vi "Main.vi"() -> ()   [LabVIEW 2022 SP3]
uses:
  <vilib>/Analysis/baseanly.llb/Mean (DBL).vi
  <vilib>/Analysis/NI_AALBase.lvlib
panel:
  in  "Calibration points":T1(array[ring])
  out "Results:":string[][](table)
  in  "Voltage [V] (max. 3.5V)":string
  in  "Confirm initialization":bool
  in  "100K FILTER":u16(ring) items=["FILTER ON", "FILTER OFF"]
  in  "IMPEDANCE [Ohm]":u16(ring) items=["50", "1M"]
  in  "COUPLING":u16(ring) items=["AC", "DC"]
  in  "counter Agilent 53131A - GPIB  [10]":string="1"
  in  "Number of measurements for each calibration point:[max 20]":i32=5
  in  "oscilloscope  Siglent SDS1102X+":refnum<visa-resource-name>="COM1"
  out "Current state:":enum16{"Init", "Measure", "Wait", "End"}(ring)
  in  "Start measuring":bool
  in  "STOP button":bool
  in  "generator Agilent 33220A":refnum<visa-resource-name>="COM1"
  # "Input settings:"
  # "Measuring:"
  # "Measurement settings:"
  # "Generator settings:"
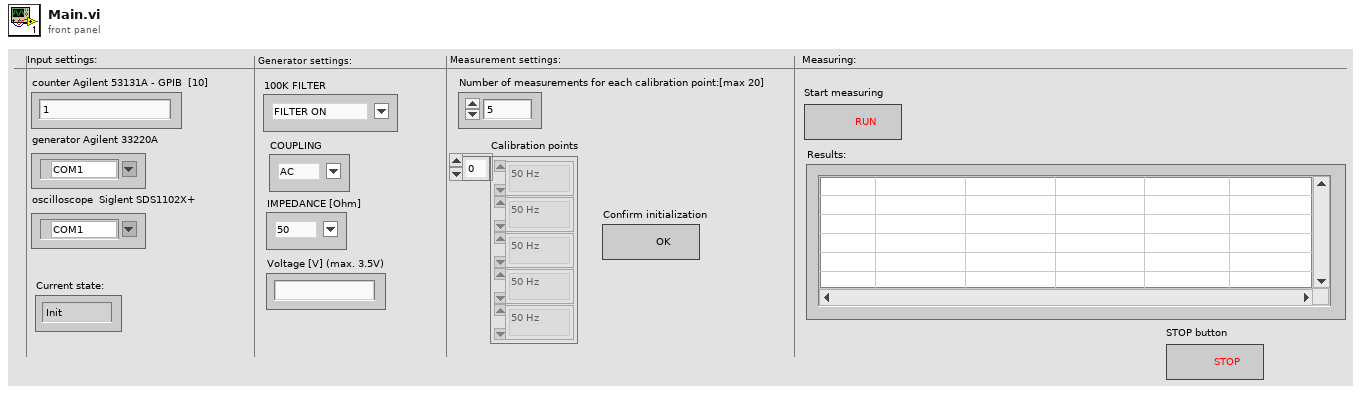
[diagram p1: front panel]
types:
  T1 = enum16{"50 Hz", "1 kHz", "5 kHz", "20 kHz", "50 kHz", "100 kHz"}[]
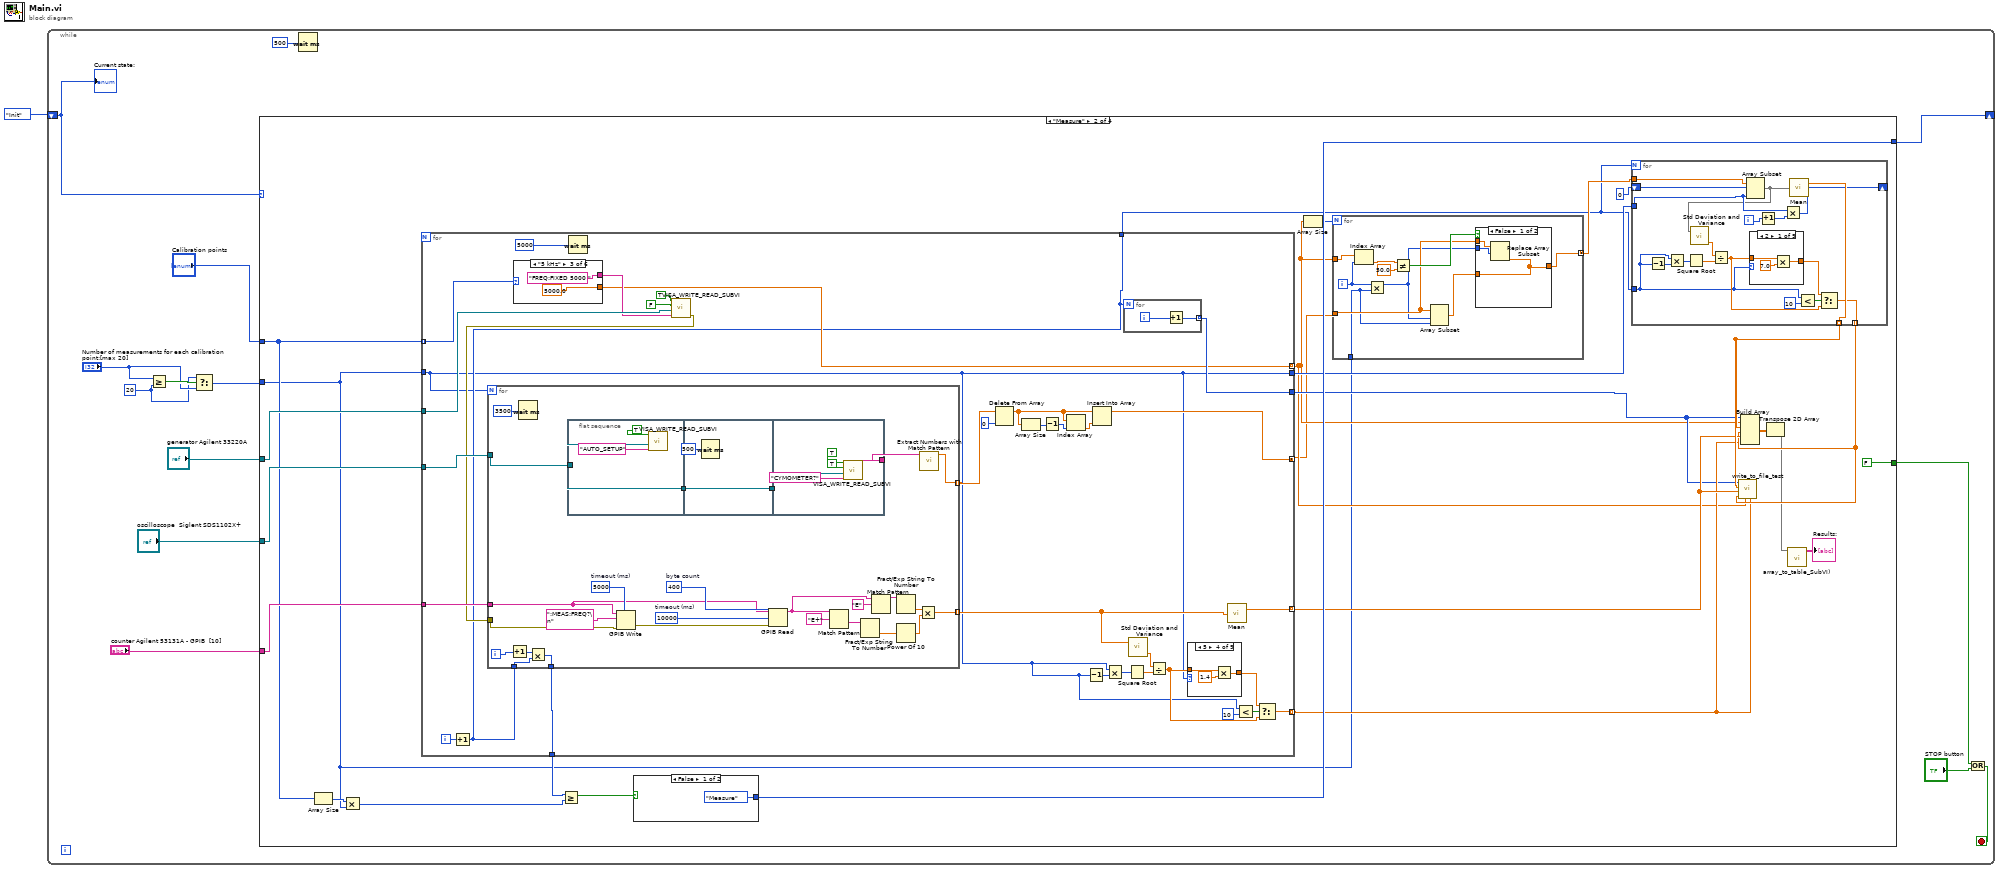
[diagram p0: block diagram]
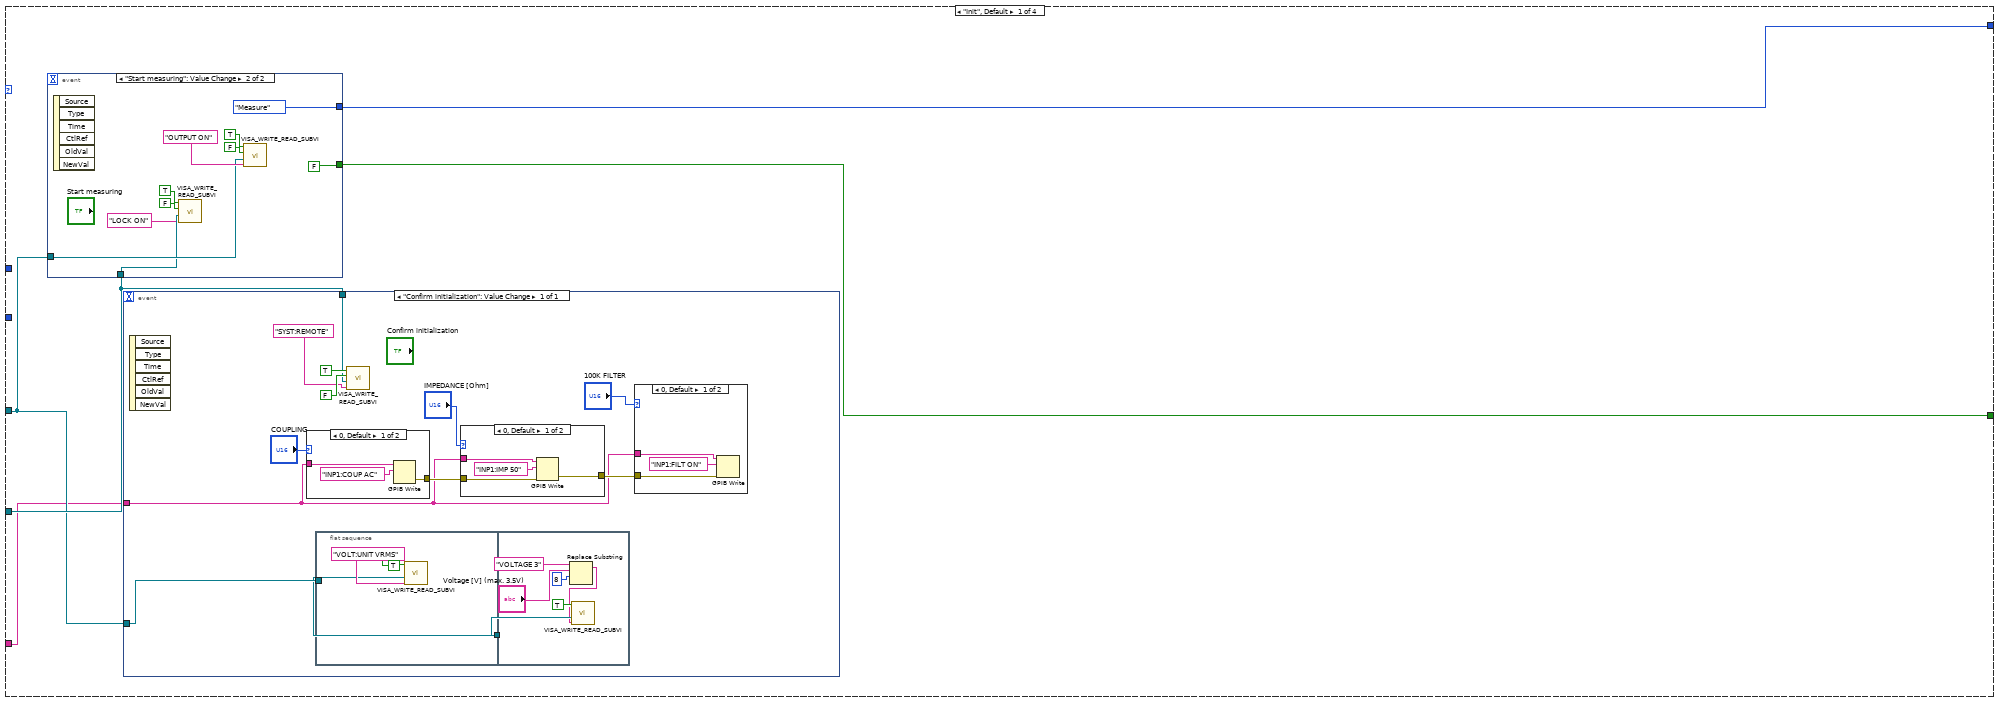
[diagram p2: hidden frame]
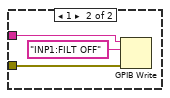
[diagram p3: hidden frame]
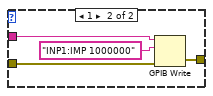
[diagram p4: hidden frame]
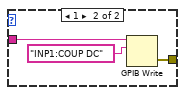
[diagram p5: hidden frame]
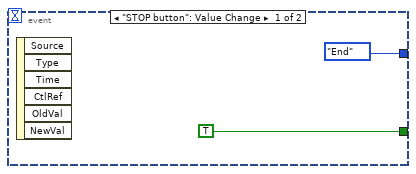
[diagram p6: hidden frame]
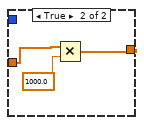
[diagram p7: hidden frame]
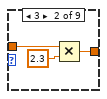
[diagram p8: hidden frame]
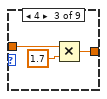
[diagram p9: hidden frame]
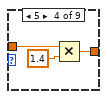
[diagram p10: hidden frame]
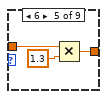
[diagram p11: hidden frame]
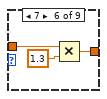
[diagram p12: hidden frame]
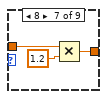
[diagram p13: hidden frame]
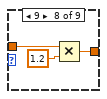
[diagram p14: hidden frame]
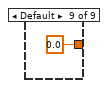
[diagram p15: hidden frame]
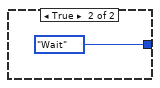
[diagram p16: hidden frame]
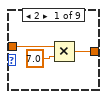
[diagram p17: hidden frame]
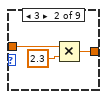
[diagram p18: hidden frame]
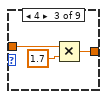
[diagram p19: hidden frame]
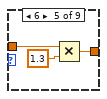
[diagram p20: hidden frame]
diagram:
  n1 = while {
    shift-right: [w4] -> _
    shift-left: enum16{"Init", "Measure", "Wait", "End"}."Init" -> [w14]
    stop <- w5 stop-if-true
    w9 = 20 ("y")
    n2 = Greater Or Equal?(x="Number of measurements for each calibration point:[max 20]", y=w9) -> (x >= y?=w11:bool)
    n3 = Select(t=w9, s=w11, f="Number of measurements for each calibration point:[max 20]") -> (s? t:f=w8:i32)
    n4 = case shown="\"Measure\"" w14 {
      tunnel: [w20 w93 enum16{"Init", "Measure", "Wait", "End"}."Init" enum16{"Init", "Measure", "Wait", "End"}."Init"] -> w4
      tunnel: [w16 FALSE ("stop") FALSE ("stop") TRUE ("stop")] -> w6
      tunnel: "generator Agilent 33220A" -> [w18 w98 _ _]
      tunnel: "Calibration points" -> [_ w95 _ _]
      tunnel: "oscilloscope  Siglent SDS1102X+" -> [w19 w97 _ _]
      tunnel: w8 -> [_ w77 _ _]
      tunnel: "counter Agilent 53131A - GPIB  [10]" -> [w17 w96 _ _]
      frame "Init", Default {
        n5 = event shown="[1] \"Start measuring\": Value Change" {
          selector: _ -> [_ _]
          dyn-events: _ -> [_ _]
          timeout: _ -> [_ _]
          tunnel: [enum16{"Init", "Measure", "Wait", "End"}."End" enum16{"Init", "Measure", "Wait", "End"}."Measure"] -> w20
          tunnel: [TRUE ("stop") FALSE ("Boolean")] -> w16
          tunnel: w18 -> [_ w71]
          tunnel: w19 -> [_ w68]
          event "STOP button": Value Change {
            n6 = event-data() -> ()  [unwired: 1 in, 6 out]
          }
          event "Start measuring": Value Change {
            n7 = event-data() -> ()  [unwired: 1 in, 6 out]
            n8 = call "VISA_WRITE_READ_SUBVI.vi"("Command"="LOCK ON", "VISA resource name"=w68, "Read 2"=FALSE ("Read"), "Write 2"=TRUE ("Write")) -> ()  [unwired: 3 in, 2 out]
            n9 = call "VISA_WRITE_READ_SUBVI.vi"("Command"="OUTPUT ON", "VISA resource name"=w71, "Read 2"=FALSE ("Read"), "Write 2"=TRUE ("Write")) -> ()  [unwired: 3 in, 2 out]
          }
        }
        n10 = event shown="[0] \"Confirm initialization\": Value Change" {
          selector: _ -> [_]
          dyn-events: _ -> [_]
          timeout: _ -> [_]
          tunnel: w19 -> [w30]
          tunnel: w18 -> [w22]
          tunnel: w17 -> [w23]
          event "Confirm initialization": Value Change {
            n11 = event-data() -> ()  [unwired: 1 in, 6 out]
            n12 = case shown="0, Default" "COUPLING" {
              tunnel: w23 -> [w58 w61]
              tunnel: [w56 w59] -> w28
              frame 0, Default {
                n13 = GPIB Write(0:w58, 1:"INP1:COUP AC" ("Command")) -> (6:w56:errorcluster)  [unwired: 3 in, 1 out]
              }
              frame 1 {
                n14 = GPIB Write(0:w61, 1:"INP1:COUP DC" ("Command")) -> (6:w59:errorcluster)  [unwired: 3 in, 1 out]
              }
            }
            n15 = flat-sequence {
              tunnel: w22 -> [w33]
              tunnel: [w33] -> w21
              tunnel: w21 -> [w40]
              frame #0 {
                n16 = call "VISA_WRITE_READ_SUBVI.vi"("Command"="VOLT:UNIT VRMS", "VISA resource name"=w33, "Write 2"=TRUE) -> ()  [unwired: 4 in, 2 out]
              }
              frame #1 {
                n17 = Replace Substring(3:8 ("offset (0)"), 4:"Voltage [V] (max. 3.5V)", 5:"VOLTAGE 3" ("Command")) -> (1:w36:string)  [unwired: 1 in, 1 out]
                n18 = call "VISA_WRITE_READ_SUBVI.vi"("Command"=w36, "VISA resource name"=w40, "Write 2"=TRUE) -> ()  [unwired: 4 in, 2 out]
              }
            }
            n19 = call "VISA_WRITE_READ_SUBVI.vi"("Command"="SYST:REMOTE", "VISA resource name"=w30, "Read 2"=FALSE ("Read"), "Write 2"=TRUE ("Write")) -> ()  [unwired: 3 in, 2 out]
            n20 = case shown="0, Default" "IMPEDANCE [Ohm]" {
              tunnel: w23 -> [w51 w53]
              tunnel: w28 -> [w49 w54]
              tunnel: [w48 w55] -> w27
              frame 0, Default {
                n21 = GPIB Write(0:w51, 1:"INP1:IMP 50" ("Command"), 3:w49) -> (6:w48:errorcluster)  [unwired: 2 in, 1 out]
              }
              frame 1 {
                n22 = GPIB Write(0:w53, 1:"INP1:IMP 1000000" ("Command"), 3:w54) -> (6:w55:errorcluster)  [unwired: 2 in, 1 out]
              }
            }
            n23 = case shown="0, Default" "100K FILTER" {
              tunnel: w23 -> [w43 w46]
              tunnel: w27 -> [w42 w45]
              frame 0, Default {
                n24 = GPIB Write(0:w43, 1:"INP1:FILT ON" ("data"), 3:w42) -> ()  [unwired: 2 in, 2 out]
              }
              frame 1 {
                n25 = GPIB Write(0:w46, 1:"INP1:FILT OFF" ("data"), 3:w45) -> ()  [unwired: 2 in, 2 out]
              }
            }
          }
        }
      }
      frame "Measure" {
        n26 = Array Size(array=w95) -> (size(s)=w94:i32)
        n27 = Multiply(x=w94, y=w77) -> (x*y=w90:i32)
        n28 = for {
          tunnel: w98 -> [w183]
          tunnel: w95 -> [w178] mode=indexing
          tunnel: w77 -> [w161]
          tunnel: w97 -> [w181]
          tunnel: w96 -> [w180]
          tunnel: [w177] -> w85 mode=indexing
          tunnel: [w175] -> w91
          tunnel: [w164] -> w79 mode=concatenating
          tunnel: [w161] -> w89
          tunnel: [w174] -> w83 mode=indexing
          tunnel: [w172] -> w80 mode=indexing
          tunnel: [w173] -> w82
          tunnel: [w163] -> w76
          i -> [w162]
          n29 = Increment(x=w162) -> (x+1=w163:i32)
          n30 = case shown="\"5 kHz\"" w178 {
            tunnel: ["FREQ:FIXED 50 " ("Command") "FREQ:FIXED 1000 " ("Command") "FREQ:FIXED 5000 " ("Command") "FREQ:FIXED 20000 " ("Command") "FREQ:FIXED 50000 " ("Command") "FREQ:FIXED 100000" ("Command")] -> w182
            tunnel: [50.0 1000.0 5000.0 20000.0 50000.0 100000.0] -> w172
            frame "50 Hz", Default {
            }
            frame "1 kHz" {
            }
            frame "5 kHz" {
            }
            frame "20 kHz" {
            }
            frame "50 kHz" {
            }
            frame "100 kHz" {
            }
          }
          n31 = Wait (ms)(milliseconds to wait=u32 5000) -> ()  [unwired: 1 out]
          n32 = call "VISA_WRITE_READ_SUBVI.vi"("Command"=w182, "VISA resource name"=w183, "Read 2"=FALSE ("Read"), "Write 2"=TRUE ("Write")) -> ("error out"=w179:errorcluster)  [unwired: 3 in, 1 out]
          n33 = for {
            N: w161 -> [_]
            tunnel: w181 -> [w196]
            tunnel: w180 -> [w216]
            tunnel: [w200] -> w171 mode=indexing
            tunnel: [w212] -> w176 mode=indexing
            tunnel: w179 -> [w215]
            tunnel: w163 -> [w207]
            tunnel: [w201] -> w175
            i -> [w206]
            w217 = 10000  # timeout (ms)
            w219 = 400  # byte count
            w218 = 5000  # timeout (ms)
            n34 = Increment(x=w206) -> (x+1=w205:i32)
            n35 = Wait (ms)(milliseconds to wait=u32 3500) -> ()  [unwired: 1 out]
            n36 = Multiply(x=w205, y=w207) -> (x*y=w201:i32)
            n37 = flat-sequence {
              tunnel: w196 -> [w222]
              tunnel: [w222] -> w198
              tunnel: w198 -> [w225]
              tunnel: [w225] -> w197
              tunnel: [w228] -> w199
              tunnel: w197 -> [w227]
              frame #0 {
                n38 = call "VISA_WRITE_READ_SUBVI.vi"("Command"="AUTO_SETUP", "VISA resource name"=w222, "Write 2"=TRUE) -> ()  [unwired: 4 in, 2 out]
              }
              frame #1 {
                n39 = Wait (ms)(milliseconds to wait=u32 500) -> ()  [unwired: 1 out]
              }
              frame #2 {
                n40 = call "VISA_WRITE_READ_SUBVI.vi"("Command"="CYMOMETER?", "VISA resource name"=w227, "Read 2"=TRUE, "Write 2"=TRUE) -> ("Response"=w228:string)  [unwired: 3 in, 1 out]
              }
            }
            n41 = GPIB Write(0:w216, 1:":MEAS:FREQ?\n" ("Characters to Write"), 3:w215, 4:w218) -> (6:w221:errorcluster)  [unwired: 1 in, 1 out]
            n42 = GPIB Read(0:w216, 1:w219, 3:w221, 4:w217) -> (5:w204:string)  [unwired: 1 in, 2 out]
            n43 = Match Pattern(string=w204, regular expression="E+") -> (after substring=w213:string)  [unwired: 1 in, 3 out]
            n44 = Fract/Exp String To Number(string=w213) -> (number=w210:dbl)  [unwired: 3 in, 1 out]
            n45 = Match Pattern(string=w204, regular expression="E") -> (before substring=w203:string)  [unwired: 1 in, 3 out]
            n46 = Fract/Exp String To Number(string=w203) -> (number=w211:dbl)  [unwired: 3 in, 1 out]
            n47 = Power Of 10(x=w210) -> (10^x=w209:dbl)
            n48 = Multiply(x=w211, y=w209) -> (x*y=w212:dbl)
            n49 = call "Extract Numbers with Match Pattern.vi"("String"=w199) -> ("Numeric"=w200:dbl)  [unwired: 10 in]
          }
          n50 = Delete From Array(array=w171, index=0) -> (array with subset deleted=w169:dbl[])  [unwired: 1 in, 1 out]
          n51 = Array Size(array=w169) -> (size(s)=w165:i32)
          n52 = Decrement(x=w165) -> (x-1=w166:i32)
          n53 = Index Array(array=w169, index=w166) -> (element=w167:dbl)
          n54 = Decrement(x=w161) -> (x-1=w192:i32)
          n55 = Insert Into Array(array=w169, new element=w167) -> (w164:dbl[])  [unwired: 1 in]
          n56 = Multiply(x=w161, y=w192) -> (x*y=w191:i32)
          n57 = for {
            N: w163 -> [_]
            tunnel: [w194] -> w173 mode=indexing
            i -> [w195]
            n58 = Increment(x=w195) -> (x+1=w194:i32)
          }
          n59 = Square Root(x=w191) -> (sqrt(x)=w190:dbl)
          n60 = call <vilib>:"Std Deviation and Variance.vi"("X"=w176) -> ("variance"=w170:dbl)  [unwired: 1 in, 2 out]
          n61 = Divide(x=w170, y=w190) -> (x/y=w187:dbl)
          n62 = case shown="5" w161 {
            tunnel: [w233 w236 w239 w242 w245 w248 w251 w254 0.0] -> w188
            tunnel: w187 -> [w232 w235 w238 w241 w244 w247 w250 w253 _]
            frame 2 {
              n63 = Multiply(x=w232, y=7.0) -> (x*y=w233:dbl)
            }
            frame 3 {
              n64 = Multiply(x=w235, y=2.3) -> (x*y=w236:dbl)
            }
            frame 4 {
              n65 = Multiply(x=w238, y=1.7) -> (x*y=w239:dbl)
            }
            frame 5 {
              n66 = Multiply(x=w241, y=1.4) -> (x*y=w242:dbl)
            }
            frame 6 {
              n67 = Multiply(x=w244, y=1.3) -> (x*y=w245:dbl)
            }
            frame 7 {
              n68 = Multiply(x=w247, y=1.3) -> (x*y=w248:dbl)
            }
            frame 8 {
              n69 = Multiply(x=w250, y=1.2) -> (x*y=w251:dbl)
            }
            frame 9 {
              n70 = Multiply(x=w253, y=1.2) -> (x*y=w254:dbl)
            }
            frame Default {
            }
          }
          n71 = call-poly <vilib>:"Mean.vi"("X"=w176) -> ("mean"=w177:dbl)  [unwired: 1 out]
          n72 = Less?(x=w161, y=10) -> (x < y?=w189:bool)
          n73 = Select(t=w188, s=w189, f=w187) -> (s? t:f=w174:dbl)
        }
        n74 = Greater Or Equal?(x=w91, y=w90) -> (x >= y?=w92:bool)
        n75 = case shown="False" w92 {
          tunnel: [enum16{"Init", "Measure", "Wait", "End"}."Measure" enum16{"Init", "Measure", "Wait", "End"}."Wait"] -> w93
          frame False {
          }
          frame True {
          }
        }
        n76 = Array Size(array=w80) -> (size(s)=w81:i32)
        n77 = for {
          N: w81 -> [_]
          tunnel: w80 -> [w109]
          tunnel: w79 -> [w103]
          tunnel: [w106] -> w78 mode=concatenating
          tunnel: w77 -> [w100]
          i -> [w102]
          n78 = Index Array(array=w109, index=w102) -> (element=w105:dbl)
          n79 = Multiply(x=w102, y=w100) -> (x*y=w101:i32)
          n80 = Not Equal?(x=w105, y=50.0) -> (x != y?=w107:bool)
          n81 = Array Subset(array=w103, index=w101, length=w100) -> (w104:dbl[])
          n82 = case shown="False" w107 {
            tunnel: [w110 w113] -> w106
            tunnel: w104 -> [w110 w114]
            tunnel: w103 -> [w112 _]
            tunnel: w101 -> [w111 _]
            frame False {
              n83 = Replace Array Subset(array=w112, new element=w110, index=w111) -> ()  [unwired: 1 out]
            }
            frame True {
              n84 = Multiply(x=w114, y=1000.0) -> (x*y=w113:dbl[])
            }
          }
        }
        n85 = for {
          N: w76 -> [_]
          tunnel: w78 -> [w118]
          tunnel: w89 -> [w131]
          shift-right: [w128] -> _
          shift-left: 0 -> [w132]
          tunnel: [w129] -> w86 mode=indexing
          tunnel: w76 -> [w119]
          tunnel: [w120] -> w84 mode=indexing
          i -> [w130]
          n86 = Decrement(x=w119) -> (x-1=w127:i32)
          n87 = Multiply(x=w119, y=w127) -> (x*y=w126:i32)
          n88 = Square Root(x=w126) -> (sqrt(x)=w125:dbl)
          n89 = Array Subset(array=w118, index=w132, length=w131) -> (w117:dbl[])
          n90 = call <vilib>:"Std Deviation and Variance.vi"("X"=w117) -> ("variance"=w116:dbl)  [unwired: 1 in, 2 out]
          n91 = Divide(x=w116, y=w125) -> (x/y=w122:dbl)
          n92 = case shown="2" w119 {
            tunnel: [w135 w138 w141 w144 w147 w150 w153 w156 0.0] -> w123
            tunnel: w122 -> [w134 w137 w140 w143 w146 w149 w152 w155 _]
            frame 2 {
              n93 = Multiply(x=w134, y=7.0) -> (x*y=w135:dbl)
            }
            frame 3 {
              n94 = Multiply(x=w137, y=2.3) -> (x*y=w138:dbl)
            }
            frame 4 {
              n95 = Multiply(x=w140, y=1.7) -> (x*y=w141:dbl)
            }
            frame 5 {
              n96 = Multiply(x=w143, y=1.4) -> (x*y=w144:dbl)
            }
            frame 6 {
              n97 = Multiply(x=w146, y=1.3) -> (x*y=w147:dbl)
            }
            frame 7 {
              n98 = Multiply(x=w149, y=1.3) -> (x*y=w150:dbl)
            }
            frame 8 {
              n99 = Multiply(x=w152, y=1.2) -> (x*y=w153:dbl)
            }
            frame 9 {
              n100 = Multiply(x=w155, y=1.2) -> (x*y=w156:dbl)
            }
            frame Default {
            }
          }
          n101 = Increment(x=w130) -> (x+1=w133:i32)
          n102 = Multiply(x=w131, y=w133) -> (x*y=w128:i32)
          n103 = call-poly <vilib>:"Mean.vi"("X"=w117) -> ("mean"=w129:dbl)  [unwired: 1 out]
          n104 = Less?(x=w119, y=10) -> (x < y?=w124:bool)
          n105 = Select(t=w123, s=w124, f=w122) -> (s? t:f=w120:dbl)
        }
        n106 = call "write_to_file_test.vi"("ua 2"=w83, "freq"=w80, "ua"=w84, "count"=w85, "osc"=w86, "n"=w82) -> ()  [unwired: 6 in]
        n107 = Build Array(w82, w80, w86, w84, w85, w83) -> (w87:dbl[][])
        n108 = Transpose 2D Array(2D array=w87) -> (transposed array=w75:dbl[][])
        n109 = call "array_to_table_SubVI).vi"("Array in"=w75) -> ("Array out"=→"Results:":string[][])  [unwired: 10 in]
      }
      frame "Wait" {
      }
      frame "End" {
      }
    }
    n110 = Wait (ms)(milliseconds to wait=u32 500) -> ()  [unwired: 1 out]
    n111 = Or(x=w6, y="STOP button") -> (x .or. y?=w5:bool)
    "Current state:" <- w14
  }
